vi "ukol3.vi"() -> ()   [LabVIEW 2023]
uses:
  <vilib>/Analysis/4window.llb/windowTd.ctl
  <vilib>/measure/maspectr.llb/FFT Spectrum (Mag-Phase) for 1 Chan.vi
  <vilib>/measure/NI_MABase.lvlib
  <vilib>/measure/NI_MAPro.lvlib
  <vilib>/Analysis/NI_AALPro.lvlib
panel:
  out "x*y":dbl
  out "max value":dbl
  in  "Array":T1[](array[typedef]) items=["Rectangle"=0, "Hanning"=1, "Hamming"=2, "Blackman-Harris"=3, "Exact Blackman"=4, "Blackman"=5, "Flat Top"=6, "4 Term B-Harris "=7, "7 Term B-Harris"=8, "Low Sidelobe"=9, "Blackman Nuttall"=11, "Triangle"=30, "Bartlett-Hanning"=31, "Bohman"=32, "Parzen"=33, "Welch"=34, "Kaiser"=60, "Dolph-Chebyshev"=61, "Gaussian"=62]
  out "XY Graph":cluster{dbl[], dbl[]}[](graph)
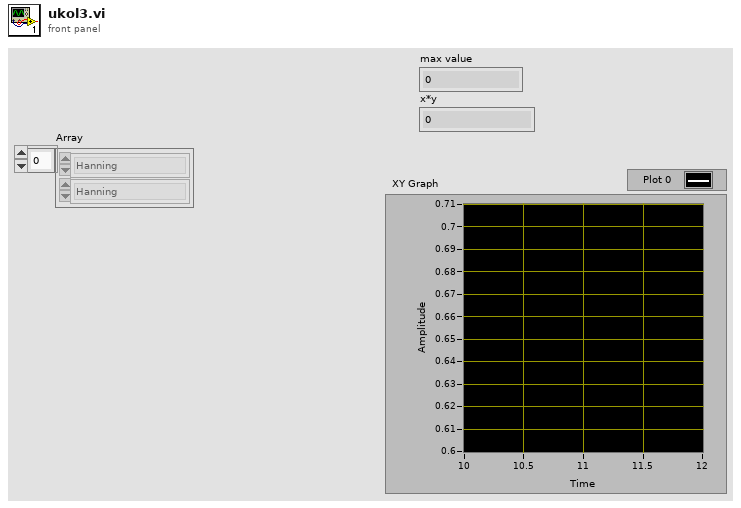
[diagram p1: front panel]
types:
  T1 = typedef "NI_AALPro.lvlib/windowTd.ctl" = u32
  T2 = cluster{"frequency":dbl, "amplitude":dbl, "phase":dbl}
  T3 = cluster{"frequency":dbl, "amplitude":dbl, "phase":dbl}[]
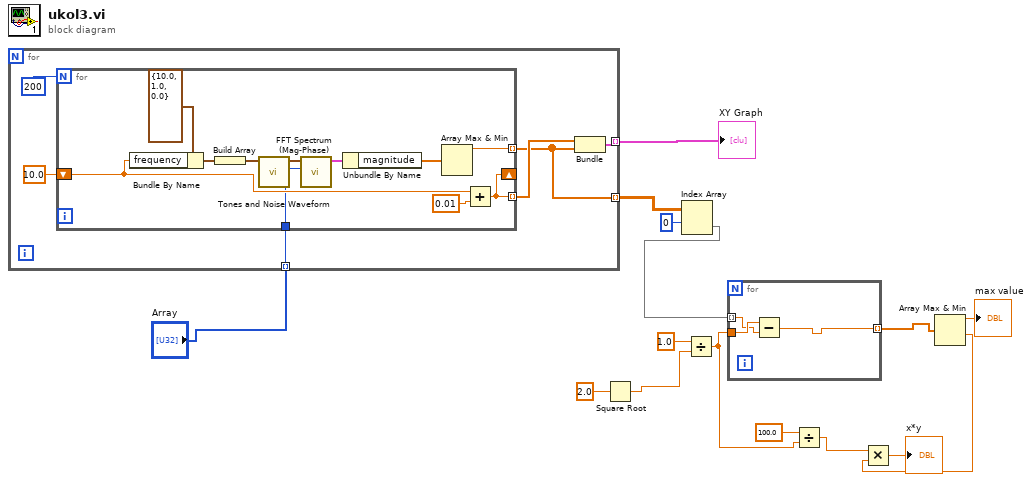
[diagram p0: block diagram]
diagram:
  n1 = for {
    tunnel: [w19] -> w15 mode=indexing
    tunnel: "Array" -> [w17] mode=indexing
    tunnel: [w16] -> w13 mode=indexing
    n2 = for {
      N: 200 -> [_]
      shift-right: [w23] -> _
      shift-left: 10.0 -> [w30]
      tunnel: [w24] -> w16 mode=indexing
      tunnel: [w23] -> w18 mode=indexing
      tunnel: w17 -> [w22]
      n3 = Bundle By Name(cluster=T2 {"frequency"=10.0, "amplitude"=1.0, "phase"=0.0}, "frequency"=w30) -> (w28:T2)
      n4 = Build Array(w28) -> (w29:T3)
      n5 = call <vilib>:"Tones and Noise Waveform.vi"("tones"=w29) -> ("signal out"=w27:waveform(dbl))  [unwired: 9 in, 1 out]
      n6 = call-poly <vilib>:"FFT Spectrum (Mag-Phase).vi"("window"=w22, "time signal"=w27) -> ("magnitude"=w26:cluster{"f0":dbl, "df":dbl, "magnitude":dbl[]})  [unwired: 5 in, 4 out]
      n7 = Unbundle By Name(w26) -> ("magnitude"=w25:dbl[])
      n8 = Array Max & Min(array=w25) -> (max value=w24:dbl)  [unwired: 3 out]
      n9 = Add(x=w30, y=0.01) -> (x+y=w23:dbl)
    }
    n10 = Bundle(w18, w16) -> (w19:cluster{dbl[], dbl[]})  [unwired: 1 in]
  }
  "XY Graph" <- w15
  n11 = Square Root(x=2.0) -> (sqrt(x)=w10:dbl)
  n12 = Index Array(array=w13, index (row)=0) -> (element=w8:dbl[])  [unwired: 1 in]
  n13 = Divide(x=1.0, y=w10) -> (x/y=w5:dbl)
  n14 = for {
    tunnel: w8 -> [w33] mode=indexing
    tunnel: w5 -> [w34]
    tunnel: [w35] -> w7 mode=indexing
    n15 = Subtract(x=w34, y=w33) -> (x-y=w35:dbl)
  }
  n16 = Divide(x=100.0, y=w5) -> (x/y=w4:dbl)
  n17 = Array Max & Min(array=w7) -> (max value=→"max value":dbl, min value=w1:dbl)  [unwired: 2 out]
  n18 = Multiply(x=w4, y=w1) -> (x*y=→"x*y":dbl)
